vi "FTW Rope design.vi"() -> ()   [LabVIEW 2013]
panel:
  in  "Look":enum16{"FTW rope"}(ring)
  out "subarray":u8[](array[numeric])
  out "colors":u32[](array[colorbox])
  out "element":u32(colorbox)
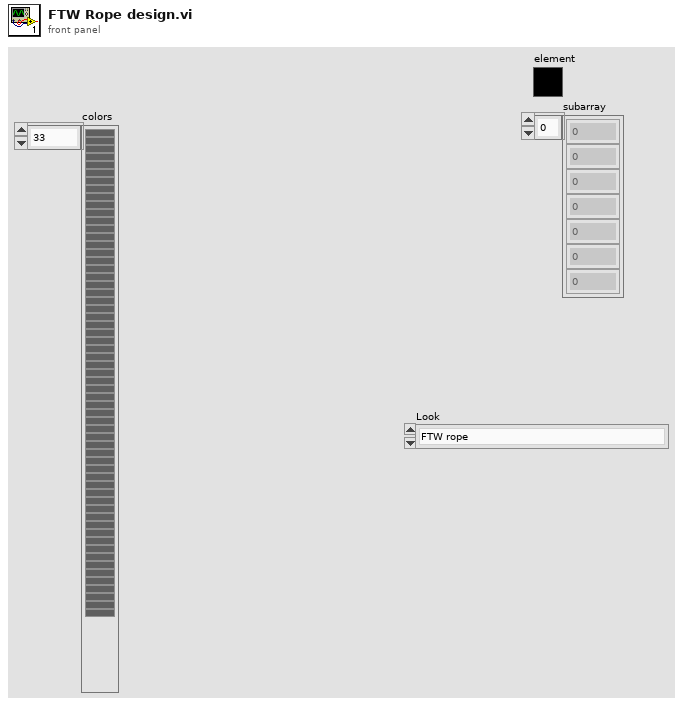
[diagram p1: front panel]
types:
  T1 = cluster{"Foreground Color":u32, "Background Color":u32, "Fill Pattern":cluster{"Row 0":u8, "Row 1":u8, "Row 2":u8, "Row 3":u8, "Row 4":u8, "Row 5":u8, "Row 6":u8, "Row 7":u8}, "Width":i16, "Mode":enum16{"Copy", "Or", "Exclusive Or", "Bit Clear", "Not Copy", "Not Or", "Nor Exclusive Or", "Not Bit Clear"}, "Style":enum32{"Solid", "Dash", "Dot", "Dash Dot", "Dash Dot Dot"}, "Fill Rule":enum32{"Even Odd", "Winding"}, "End Caps":enum32{"Default", "Flat"}}[]
  T2 = typedef "imagedata.ctl" = cluster{"image type":i32, "image depth":i32, "image":u8[], "mask":u8[], "colors":u32[], "Rectangle":cluster{"left":i16, "top":i16, "right":i16, "bottom":i16}}
  T3 = cluster{"left":i16, "top":i16, "right":i16, "bottom":i16}
  T4 = cluster{"Foreground Color":u32, "Background Color":u32, "Fill Pattern":cluster{"Row 0":u8, "Row 1":u8, "Row 2":u8, "Row 3":u8, "Row 4":u8, "Row 5":u8, "Row 6":u8, "Row 7":u8}, "Width":i16, "Mode":enum16{"Copy", "Or", "Exclusive Or", "Bit Clear", "Not Copy", "Not Or", "Nor Exclusive Or", "Not Bit Clear"}, "Style":enum32{"Solid", "Dash", "Dot", "Dash Dot", "Dash Dot Dot"}, "Fill Rule":enum32{"Even Odd", "Winding"}, "End Caps":enum32{"Default", "Flat"}}
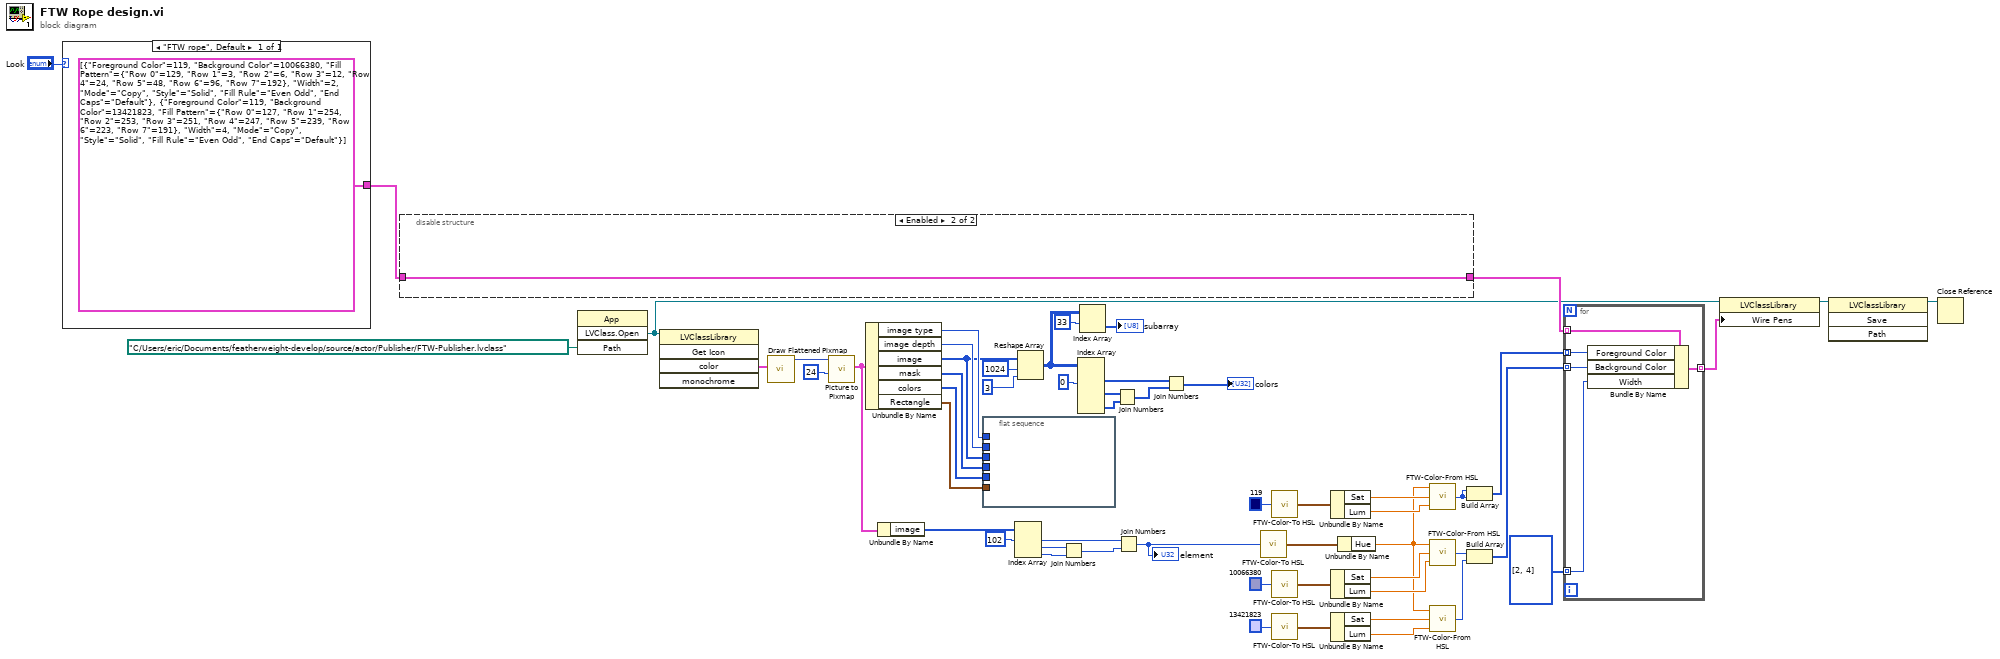
[diagram p0: block diagram]
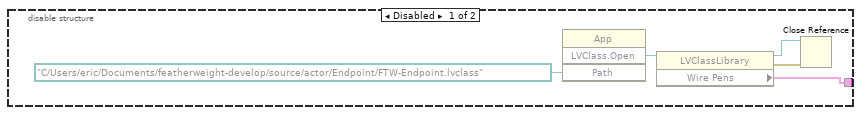
[diagram p2: hidden frame]
diagram:
  n1 = case shown="\"FTW rope\", Default" "Look" {
    tunnel: [T1 [{"Foreground Color"=119, "Background Color"=10066380, "Fill Pattern"={"Row 0"=129, "Row 1"=3, "Row 2"=6, "Row 3"=12, "Row 4"=24, "Row 5"=48, "Row 6"=96, "Row 7"=192}, "Width"=2, "Mode"=enum."Copy", "Style"=enum."Solid", "Fill Rule"=enum."Even Odd", "End Caps"=enum."Default"}, {"Foreground Color"=119, "Background Color"=13421823, "Fill Pattern"={"Row 0"=127, "Row 1"=254, "Row 2"=253, "Row 3"=251, "Row 4"=247, "Row 5"=239, "Row 6"=223, "Row 7"=191}, "Width"=4, "Mode"=enum."Copy", "Style"=enum."Solid", "Fill Rule"=enum."Even Odd", "End Caps"=enum."Default"}] ("Array")] -> w1
    frame "FTW rope", Default {
    }
  }
  n2 = disable-structure shown="Enabled" {
    disable-tunnel: [w60 w63] -> w56
    disable-tunnel: w1 -> [_ w63]
    frame Disabled {
      n3 = invoke class="App" method="LVClass.Open"("Path"=path "C:/Users/eric/Documents/featherweight-develop/source/actor/Endpoint/FTW-Endpoint.lvclass") -> ("LVClass.Open"=w61:refnum<vi>)  [unwired: 3 in, 3 out]
      n4 = property class="LVClassLibrary"(reference=w61) -> (reference out=w58:refnum<vi>, error out=w59:errorcluster, "Wire Pens"=w60:T1)  [unwired: 1 in]
      n5 = Close Reference(reference=w58, error in (no error)=w59) -> ()  [unwired: 1 out]
    }
    frame Enabled {
    }
  }
  n6 = invoke class="App" method="LVClass.Open"("Path"=path "C:/Users/eric/Documents/featherweight-develop/source/actor/Publisher/FTW-Publisher.lvclass") -> ("LVClass.Open"=w30:refnum<vi>)  [unwired: 3 in, 3 out]
  n7 = invoke class="LVClassLibrary" method="Get Icon"(reference=w30) -> ("color"=w29:T2)  [unwired: 4 in, 4 out]
  n8 = call <vilib>:"Draw Flattened Pixmap.vi"("image data"=w29) -> ("new picture"=w28:picture)  [unwired: 8 in]
  n9 = call <vilib>:"Picture to Pixmap.vi"("depth"=24, "picture"=w28) -> ("image data"=w4:T2)  [unwired: 8 in, 1 out]
  n10 = Unbundle By Name(w4) -> ("image type"=w26:i32, "image depth"=w25:i32, "image"=w21:u8[], "mask"=w24:u8[], "colors"=w23:u32[], "Rectangle"=w22:T3)
  n11 = Unbundle By Name(w4) -> ("image"=w8:u8[])
  n12 = flat-sequence {
    tunnel: w21 -> [_]
    tunnel: w26 -> [_]
    tunnel: w25 -> [_]
    tunnel: w24 -> [_]
    tunnel: w23 -> [_]
    tunnel: w22 -> [_]
    frame #0 {
    }
  }
  n13 = Index Array(array=w8, index #1=102 ("index")) -> (element #1=w12:u8, element #2=w10:u8, element #3=w9:u8)  [unwired: 2 in]
  n14 = Reshape Array(w21, 1024 ("dimension size"), 3 ("dimension size")) -> (w6:u8[][])
  n15 = Join Numbers(hi=w10, lo=w9) -> ((hi.lo)=w11:u16)
  n16 = Index Array(array=w6, index (col) #1=0 ("disabled index (col)")) -> (element #1=w14:u8[], element #2=w16:u8[], element #3=w17:u8[])  [unwired: 5 in]
  n17 = Index Array(array=w6, index (row)=33 ("index")) -> (element=→"subarray":u8[])  [unwired: 1 in]
  n18 = Join Numbers(hi=w16, lo=w17) -> ((hi.lo)=w15:u16[])
  n19 = Join Numbers(hi=w12, lo=w11) -> ((hi.lo)=w3:u32)
  "element" <- w3
  n20 = Join Numbers(hi=w14, lo=w15) -> ((hi.lo)=→"colors":u32[])
  n21 = call "FTW-Color-To HSL.vi"("Color"=w3) -> ("HSL"=w46:cluster{"Hue":dbl, "Sat":dbl, "Lum":dbl})
  n22 = call "FTW-Color-To HSL.vi"("Color"=u32 119 ("Foreground Color")) -> ("HSL"=w47:cluster{"Hue":dbl, "Sat":dbl, "Lum":dbl})
  n23 = call "FTW-Color-To HSL.vi"("Color"=u32 10066380 ("Background Color")) -> ("HSL"=w35:cluster{"Hue":dbl, "Sat":dbl, "Lum":dbl})
  n24 = call "FTW-Color-To HSL.vi"("Color"=u32 13421823 ("Background Color")) -> ("HSL"=w38:cluster{"Hue":dbl, "Sat":dbl, "Lum":dbl})
  n25 = Unbundle By Name(w47) -> ("Sat"=w45:dbl, "Lum"=w44:dbl)
  n26 = Unbundle By Name(w35) -> ("Sat"=w34:dbl, "Lum"=w33:dbl)
  n27 = Unbundle By Name(w38) -> ("Sat"=w37:dbl, "Lum"=w36:dbl)
  n28 = Unbundle By Name(w46) -> ("Hue"=w32:dbl)
  n29 = call "FTW-Color-From HSL.vi"("Luminance"=w44, "Saturation"=w45, "Hue"=w32) -> ("Color"=w43:u32)
  n30 = call "FTW-Color-From HSL.vi"("Luminance"=w33, "Saturation"=w34, "Hue"=w32) -> ("Color"=w41:u32)
  n31 = call "FTW-Color-From HSL.vi"("Luminance"=w36, "Saturation"=w37, "Hue"=w32) -> ("Color"=w40:u32)
  n32 = Build Array(w43, w43) -> (w42:u32[])
  n33 = Build Array(w41, w40) -> (w39:u32[])
  n34 = for {
    tunnel: w56 -> [w68] mode=indexing
    tunnel: i16[] [2, 4] -> [w67] mode=indexing
    tunnel: [w66] -> w53 mode=indexing
    tunnel: w42 -> [w65] mode=indexing
    tunnel: w39 -> [w64] mode=indexing
    n35 = Bundle By Name(cluster=w68, "Foreground Color"=w65, "Background Color"=w64, "Width"=w67) -> (w66:T4)
  }
  n36 = property class="LVClassLibrary"(reference=w30, "Wire Pens"=w53) -> (reference out=w52:refnum<vi>)  [unwired: 1 in, 1 out]
  n37 = invoke class="LVClassLibrary" method="Save"(reference=w52) -> (reference out=w51:refnum<vi>)  [unwired: 3 in, 3 out]
  n38 = Close Reference(reference=w51) -> ()  [unwired: 1 in, 1 out]
